vi "PXI Globals.vi"() -> ()   [LabVIEW 2020]
uses:
  Type Defs/Task Struct.ctl
  Type Defs/Channel Struct.ctl
  Type Defs/Ramping Params.ctl
  Type Defs/Counter Params.ctl
  Type Defs/DI Channel Struct.ctl
  Type Defs/PXI-AI Transfer Mode.ctl
panel:
  out "Hold outputs":bool
  out "External Start":bool
  out "UseAOQueue":bool
  out "Abort AO":bool
  out "PauseDAQ":bool
  in  "Shaker Vmax":dbl=5.0
  out "AI Data Bank Fresh":bool
  in  "AI Transfer Mode":T1
  out "DO Buffer Rewrite":bool
  out "DO Sig Bank Fresh":bool
  out "DO Config":bool
  in  "DO Sample Rate":dbl
  in  "DO BufferSize":i32
  in  "DO Channel Spec":T2
  in  "DI Sample Rate":dbl
  in  "DI BufferSize":i32
  in  "DI Channel Spec":T2
  in  "DI Tasks":T3[](array[typedef])=[{"Task name"="AI01", "Task"="", "Dual-channel task?"=FALSE, "Regenerate?"=FALSE, "Clear?"=FALSE}]
  out "DI Config":bool
  in  "VDAC":dbl=10.0
  in  "Data port":u16=4914
  out "Counter Parameters":T4={"Counter"="PXI1Slot4/ctr0", "Hi ticks"=5, "Low ticks"=4995, "Idle state"=10214, "Delay ticks"=0} {"Idle state" items=["High"=10192, "Low"=10214]; "Low ticks" max=1}
  in  "Skip Samples":i32
  out "Single precision?":bool
  out "Send Data":bool
  out "Counter Config":bool
  out "Counter Clear Task":bool
  out "AI Clear Tasks":bool
  out "Double Buffer?":bool
  in  "Num Extra Buffers":i32
  in  "Max Presentations":i32
  out "External Trigger":bool
  out "AO Config":bool
  out "Bypass NEB":bool
  out "Stop on MaxPresentations":bool
  in  "Reload Signal Bank":enum32{"OFF", "ENABLED", "FORCED"}(radio)
  out "Sig Bank Ready For Read":bool
  out "TCPData":bool
  out "AO Clear Tasks":bool
  out "AI Config":bool
  out "AO Buffer ReWrite":bool
  in  "AI Sample Rate":dbl
  in  "AO Sample Rate":dbl
  out "Auto ramping?":bool
  in  "Ramping":T5={"Ramp up?"=FALSE, "Ramp down?"=FALSE, "Ramp duration (msecs)"=0.005, "Ramp type"=enum."Cos2"}
  out "Abort Send Data Queue":bool
  out "AO Range Changed":bool
  out "Abort VmaxVmin  Notifier":bool
  out "Enable VmaxVmin Autorange":bool
  out "sweep freq":bool
  out "Stop Button Monitor":bool
  out "Abort":bool
  out "DAQ in Progress":bool
  out "StopDAQ":bool
  in  "AI BufferSize":i32
  in  "AI Channel Spec":T6[](array[typedef]) {"Terminal configuration" items=["Default"=-1, "RSE"=10083, "Differential"=10106, "Pseudodifferential"=12529]}
  in  "AO BufferSize":i32
  in  "AO Channel Spec":T6[](array[typedef]) {"Terminal configuration" items=["Default"=-1, "RSE"=10083, "Differential"=10106, "Pseudodifferential"=12529]}
  in  "STATUS port":u16=4917
  in  "Primary port":u16=4913
  in  "Client":string="169.254.59.145"
  in  "Server":string="169.254.92.87"
  in  "AI Gains":dbl[](array[numeric])
  in  "PXI DAQ Version":string="V2.0.0"
  out "sync source":tag
  in  "AO Gain (Property Node)":dbl[](array[slide])=[0.0, -3.1086244689504383e-15, 0.0, -1.7763568394002505e-15, 0.0, 0.0, 0.0, 0.0, 0.0, 0.0] min=-40.0 max=0.0 step=20.0 scale format="%#_2g"
  in  "AO voltage amplitude ( Vp)":dbl[](array[numeric])=[1.0, 1.0, 1.0, 1.0, 1.0, 1.0, 1.0, 1.0, 1.0, 1.0, 1.0] format="%_4f"
  in  "AO delay  (sec)":dbl=inf
  out "PXI error":errorcluster
  out "ButtonsPressed":bool[](array[boolean])
  in  "Counter Task":T3={"Task name"="Counter", "Task"="", "Dual-channel task?"=FALSE, "Regenerate?"=FALSE, "Clear?"=FALSE}
  in  "AI Tasks":T3[](array[typedef])=[{"Task name"="AI01", "Task"="", "Dual-channel task?"=FALSE, "Regenerate?"=FALSE, "Clear?"=FALSE}]
  in  "AO Tasks":T3[](array[typedef])=[{"Task name"="AO02", "Task"="", "Dual-channel task?"=FALSE, "Regenerate?"=FALSE, "Clear?"=FALSE}]
  # "Status"
  # "Configuration"
  # "TCP Params"
  # "1"
  # "2"
  # "3"
  # "4"
  # "5"
  # "6"
  # "7"
  # "8"
  # "9"
  # "10"
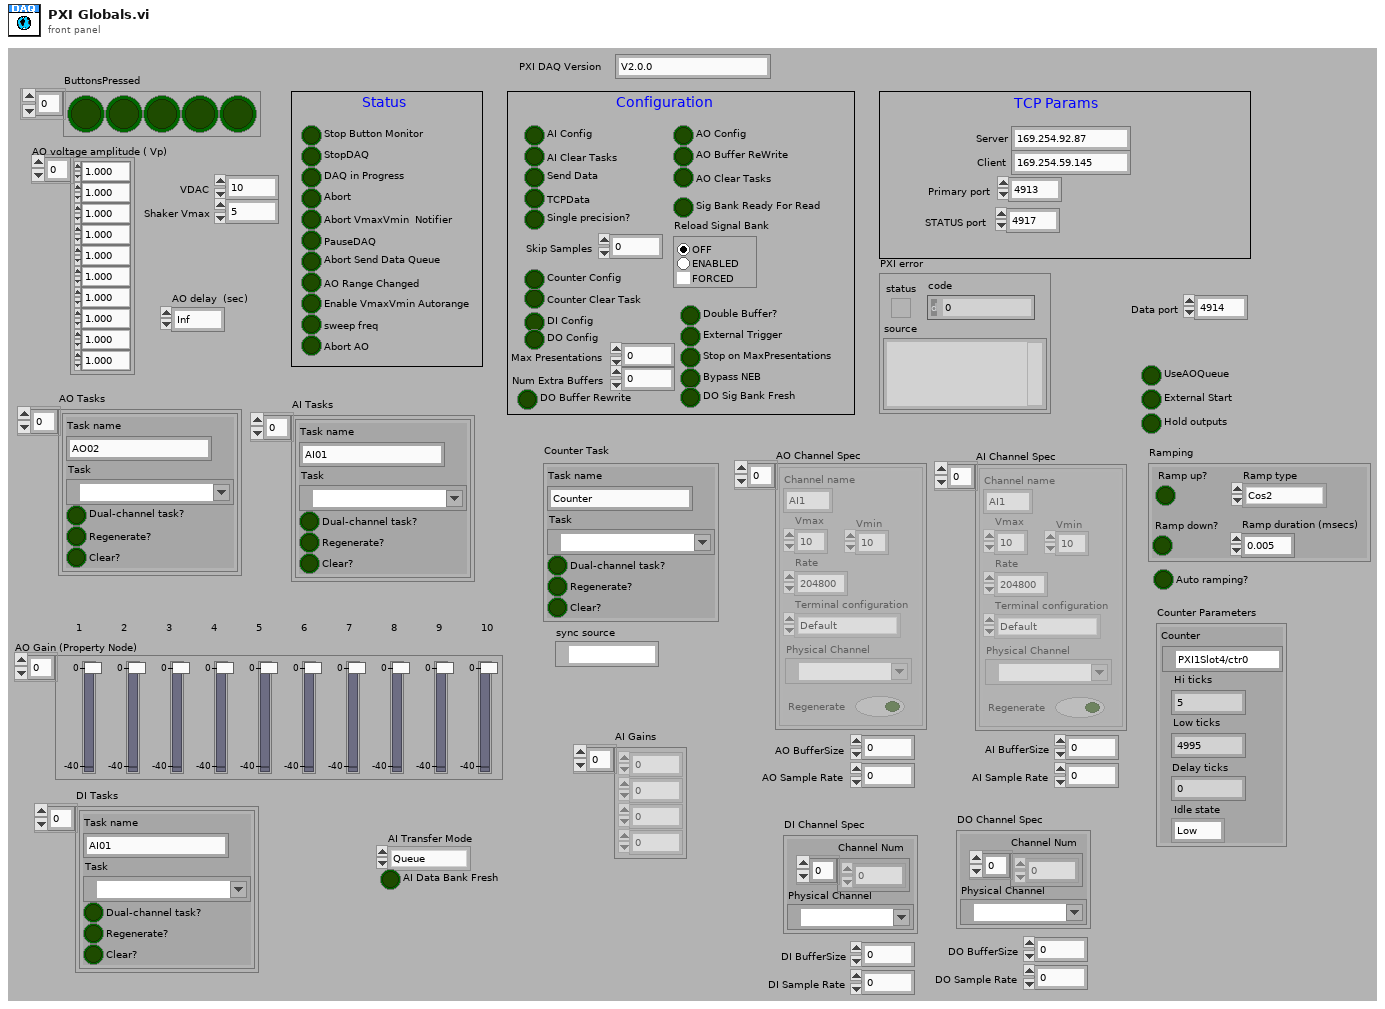
[diagram p1: front panel]
types:
  T1 = typedef "PXI-AI Transfer Mode.ctl" = enum16{"Queue", "Data Bank", "No Transfer"}
  T2 = typedef "DI Channel Struct.ctl" = cluster{"Physical Channel":tag, "Channel Num":i32[]}
  T3 = typedef "Task Struct.ctl" = cluster{"Task name":string, "Task":refnum<k21>, "Dual-channel task?":bool, "Regenerate?":bool, "Clear?":bool}
  T4 = typedef "Counter Params.ctl" = cluster{"Counter":tag, "Hi ticks":u32, "Low ticks":u32, "Idle state":i32, "Delay ticks":u32}
  T5 = typedef "Ramping Params.ctl" = cluster{"Ramp up?":bool, "Ramp down?":bool, "Ramp duration (msecs)":dbl, "Ramp type":enum16{"Linear", "Cos2"}}
  T6 = typedef "Channel Struct.ctl" = cluster{"Channel name":string, "Vmax":dbl, "Vmin":dbl, "Rate":dbl, "Terminal configuration":i32, "Physical Channel":tag, "Regenerate":bool}
diagram:
